vi "C4Dev_getBuffer.vi"(0 "c4dev in":refnum<k24>, 11 "error in (no error)":errorcluster, 12 "timeout_ms in":i64=10000) -> (4 "c4dev out":refnum<k24>, 6 "c4buf out":refnum<k24>, 15 "error out":errorcluster)   [LabVIEW 2015, in "libC4HdlLV.lvlib"]
uses:
  libC4HdlLV.lvlib
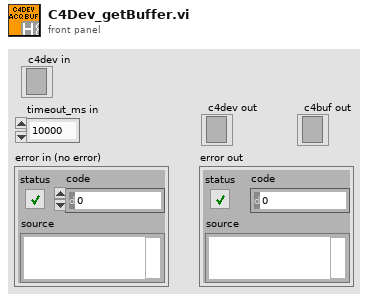
[diagram p1: front panel]
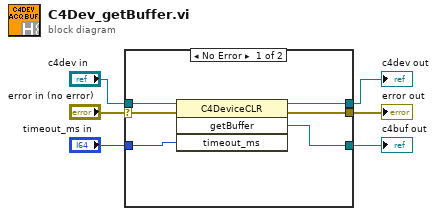
[diagram p0: block diagram]
diagram:
  n1 = case shown="No Error" "error in (no error)" {
    selector: "error in (no error)" -> [w10 w14]
    tunnel: "c4dev in" -> [w12 w13]
    tunnel: [w8 w13] -> w2
    tunnel: [w9 w14] -> w6
    tunnel: "timeout_ms in" -> [w11 _]
    tunnel: [w7 _] -> w1
    frame No Error {
      n2 = invoke class="C4DeviceCLR" method="getBuffer"(reference=w12, error in=w10, "timeout_ms"=w11) -> (reference out=w8:refnum<k24>, error out=w9:errorcluster, "getBuffer"=w7:refnum<k24>)  [unwired: 1 in, 1 out]
    }
    frame Error {
    }
  }
  "error out" <- w6
  "c4dev out" <- w2
  "c4buf out" <- w1
